vi "calcolo scostamenti QrefHref.vi"(8 "Htot ref":dbl, 9 "Q ref":dbl, 10 "Q [UM]":dbl, 11 "Htot":dbl) -> (2 "scostamento H":dbl, 3 "scostaemento Q":dbl)   [LabVIEW 2019]
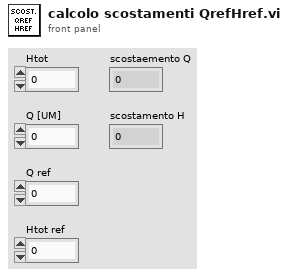
[diagram p1: front panel]
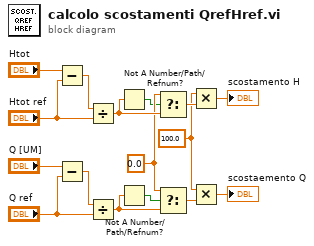
[diagram p0: block diagram]
diagram:
  w13 = 0.0 ("t")
  w6 = 100.0 ("x")
  n1 = Subtract(x="Htot", y="Htot ref") -> (x-y=w2:dbl)
  n2 = Subtract(x="Q [UM]", y="Q ref") -> (x-y=w1:dbl)
  n3 = Divide(x=w2, y="Htot ref") -> (x/y=w14:dbl)
  n4 = Divide(x=w1, y="Q ref") -> (x/y=w11:dbl)
  n5 = Not A Number/Path/Refnum?(number/path/refnum=w14) -> (NaN/Path/Refnum?=w12:bool)
  n6 = Not A Number/Path/Refnum?(number/path/refnum=w11) -> (NaN/Path/Refnum?=w10:bool)
  n7 = Select(t=w13, s=w12, f=w14) -> (s? t:f=w15:dbl)
  n8 = Select(t=w13, s=w10, f=w11) -> (s? t:f=w16:dbl)
  n9 = Multiply(x=w6, y=w15) -> (x*y=→"scostamento H":dbl)
  n10 = Multiply(x=w6, y=w16) -> (x*y=→"scostaemento Q":dbl)
